vi "Parse Command Frame.vi"(8 "error in (no error)":errorcluster, 11 "command frame":string) -> (0 "error out":errorcluster, 1 "frame valid?":bool, 2 "extended frame data":string, 3 "command":T1=3 format="%04b" items=["Turn off Transmission of Data Frame"=1, "Turn on Transmission of Data Frame"=2, "Send Header Frame"=3, "Send CFG-1 Frame"=4, "Send CFG-2 Frame"=5, "Send CFG-3 Frame"=6, "Extended Frame"=8], 5 "ID code":u16)   [LabVIEW 2015, in "NI_EP_PMU.lvlib"]
doc: "Parses command frames from a phasor data concentrator (PDC) as defined in IEEE Std C37.118.2-2011."
uses:
  <vilib>/addons/Electrical Power/PMU/NI_EP_PMU.lvlib
  <vilib>/addons/Electrical Power/PMU/Common/Controls/pmu_Command.ctl
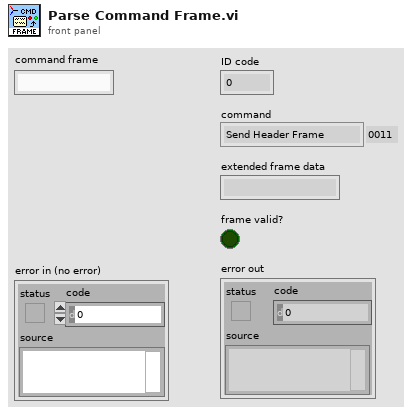
[diagram p1: front panel]
types:
  T1 = typedef "NI_EP_PMU.lvlib/pmu_Command.ctl" = u16
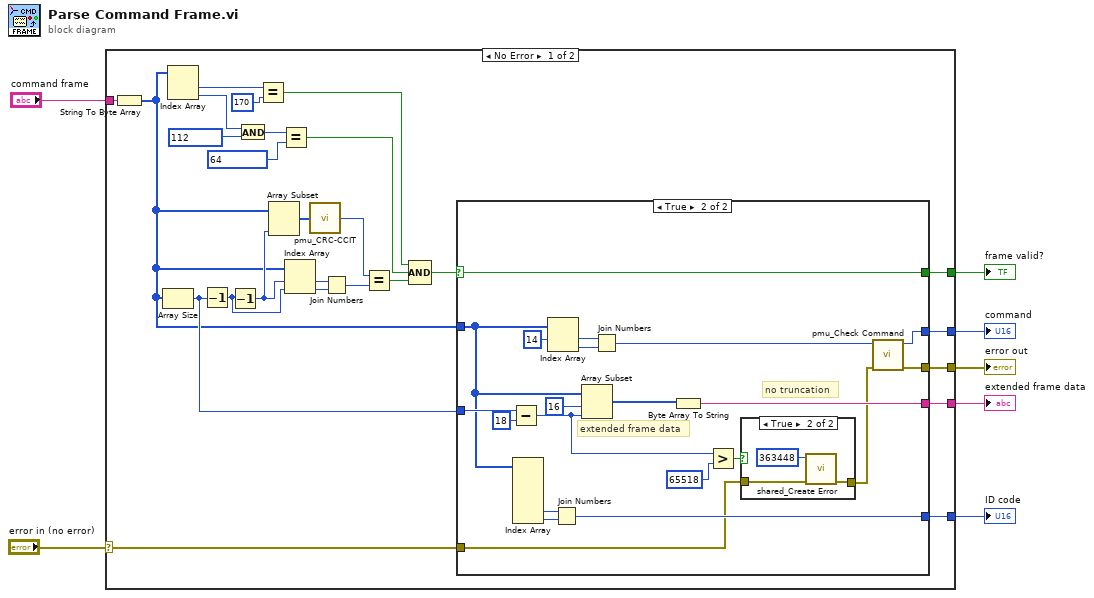
[diagram p0: block diagram]
diagram:
  n1 = case shown="No Error" "error in (no error)" {
    selector: "error in (no error)" -> [w16 w61]
    tunnel: "command frame" -> [w33 _]
    tunnel: [w24 _] -> w6
    tunnel: [w23 _] -> w5
    tunnel: [w17 w61] -> w4
    tunnel: [w19 _] -> w2
    tunnel: [w18 _] -> w1
    frame No Error {
      n2 = String To Byte Array(string=w33) -> (unsigned byte array=w13:u8[])
      n3 = Array Size(array=w13) -> (size(s)=w22:i32)
      n4 = Index Array(array=w13) -> (element #1=w32:u8, element #2=w12:u8)  [unwired: 2 in]
      n5 = Decrement(x=w22) -> (x-1=w15:i32)
      n6 = Decrement(x=w15) -> (x-1=w21:i32)
      n7 = And(x=w12, y=u8 112) -> (x .and. y?=w11:u8)
      n8 = Equal?(x=w32, y=u8 170) -> (x = y?=w9:bool)
      n9 = Array Subset(array=w13, length=w21) -> (w20:u8[])  [unwired: 1 in]
      n10 = Equal?(x=w11, y=u8 64) -> (x = y?=w8:bool)
      n11 = Index Array(array=w13, index #1=w21, index #2=w15) -> (element #1=w29:u8, element #2=w30:u8)
      n12 = call <vilib>:"pmu_CRC-CCIT.vi"("byte array"=w20) -> ("CRC-CCIT"=w27:u16)  [unwired: 13 in, 1 out]
      n13 = Join Numbers(hi=w29, lo=w30) -> ((hi.lo)=w28:u16)
      n14 = Equal?(x=w27, y=w28) -> (x = y?=w26:bool)
      n15 = Compound Arithmetic op=AND(w9, w8, w26) -> (w25:bool)
      n16 = case shown="True" w25 {
        selector: w25 -> [w35 w56]
        tunnel: [w35 w56] -> w24
        tunnel: w13 -> [_ w50]
        tunnel: [_ w52] -> w23
        tunnel: w22 -> [_ w51]
        tunnel: [_ w45] -> w19
        tunnel: [_ w36] -> w18
        tunnel: [w34 w37] -> w17
        tunnel: w16 -> [w34 w43]
        frame False {
        }
        frame True {
          # "no truncation"
          # "extended frame data"
          n17 = Subtract(x=w51, y=18) -> (x-y=w42:i32)
          n18 = Index Array(array=w50) -> (element #5=w49:u8, element #6=w48:u8)  [unwired: 6 in, 4 out]
          n19 = Index Array(array=w50, index #1=14 ("index")) -> (element #1=w40:u8, element #2=w41:u8)  [unwired: 1 in]
          n20 = Join Numbers(hi=w49, lo=w48) -> ((hi.lo)=w45:u16)
          n21 = Array Subset(array=w50, index=16, length=w42) -> (w47:u8[])
          n22 = Join Numbers(hi=w40, lo=w41) -> ((hi.lo)=w39:u16)
          n23 = Byte Array To String(unsigned byte array=w47) -> (string=w52:string)
          n24 = Greater?(x=w42, y=65518) -> (0:w44:bool)
          n25 = case shown="True" w44 {
            tunnel: [w57 w60] -> w38
            tunnel: w43 -> [w57 w59]
            frame False {
            }
            frame True {
              n26 = call <vilib>:"shared_Create Error.vi"("error in (no error)"=w59, "error code (0)"=363448) -> ("error out"=w60:errorcluster)  [unwired: 9 in]
            }
          }
          n27 = call <vilib>:"pmu_Check Command.vi"("error in (no error)"=w38, "command in"=w39) -> ("error out"=w37:errorcluster, "command out"=w36:u16)  [unwired: 8 in]
        }
      }
    }
    frame Error {
    }
  }
  "frame valid?" <- w6
  "extended frame data" <- w5
  "error out" <- w4
  "ID code" <- w2
  "command" <- w1
